vi "_layoutVirtual.vi"(0 "reference":refnum<class "SequenceDiagramGraph.lvclass">, 1 "graphics":refnum<class "Graphics.lvclass">, 2 "grid":refnum<class "Grid.lvclass">, 5 "error in (no error)":errorcluster) -> (14 "reference out":refnum<class "SequenceDiagramGraph.lvclass">, 19 "error out":errorcluster)   [LabVIEW 2012, in "SequenceDiagramGraph.lvclass"]
doc: "public void layoutVirtual(Graphics2D g2, Grid grid)"
uses:
  <resource>/Framework/Providers/Open_GDS/UML/SequenceDiagramGraph_class/SequenceDiagramGraph.lvclass
  <resource>/Framework/Providers/Open_GDS/UML/Graphics_class/Graphics.lvclass
  <resource>/Framework/Providers/Open_GDS/UML/Grid_class/Grid.lvclass
  <resource>/Framework/Providers/Open_GDS/UML/CallNode_class/CallNode.lvclass
  <resource>/Framework/Providers/Open_GDS/UML/AbstractNode_class/AbstractNode.lvclass
  <resource>/Framework/Providers/Open_GDS/UML/AbstractEdge_class/AbstractEdge.lvclass
  <resource>/Framework/Providers/Open_GDS/UML/CallEdge_class/CallEdge.lvclass
  <resource>/Framework/Providers/Open_GDS/UML/ImplicitParameterNode_class/ImplicitParameterNode.lvclass
  <resource>/Framework/Providers/Open_GDS/UML/RectangularNode_class/RectangularNode.lvclass
  <resource>/Framework/Providers/Open_GDS/UML/Graph_class/Graph.lvclass
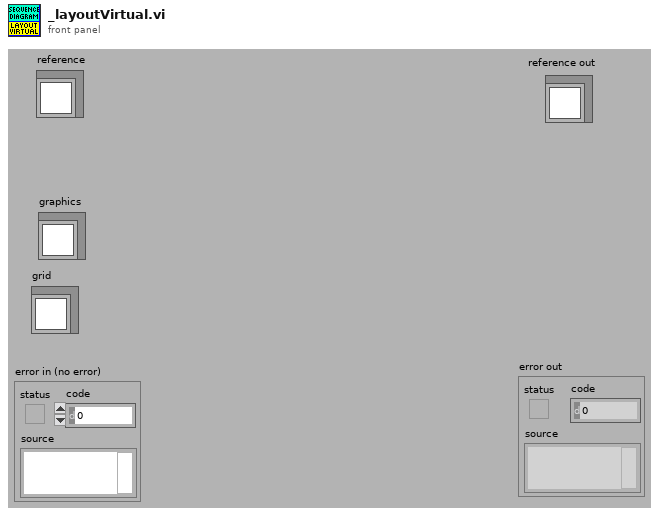
[diagram p1: front panel]
types:
  T1 = typedef "SequenceDiagramGraph.lvclass/ObjectAttributes.ctl" = cluster{"Base class":T2, "none":bool}
  T2 = typedef "Graph.lvclass/ObjectAttributes.ctl" = cluster{"nodes":refnum<class "AbstractNode.lvclass">[], "edges":refnum<class "AbstractEdge.lvclass">[], "nodesToBeRemoved":refnum<class "AbstractNode.lvclass">[], "edgesToBeRemoved":refnum<class "AbstractEdge.lvclass">[], "needsLayout":bool, "LayoutNodes":refnum<class "AbstractNode.lvclass">[]}
  T3 = typedef "Rectangle Rectangle2D.ctl" = cluster{"x":dbl, "y":dbl, "width":dbl, "height":dbl}
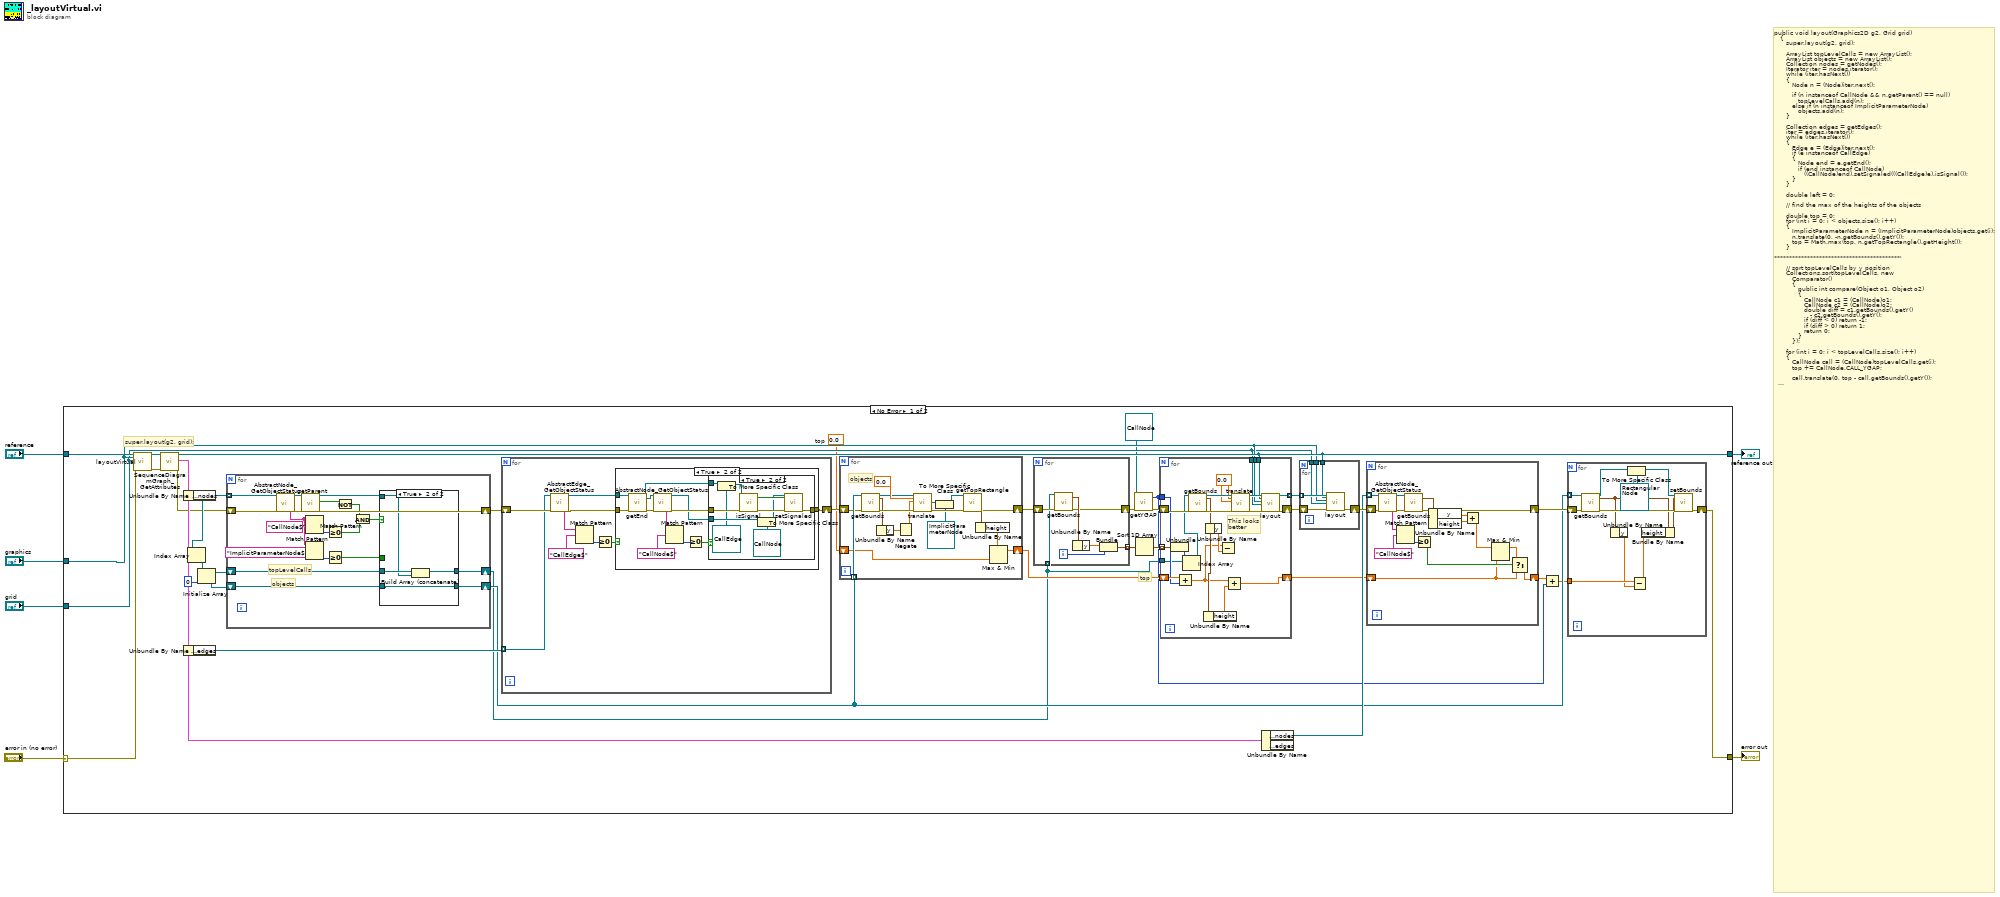
[diagram p0: block diagram]
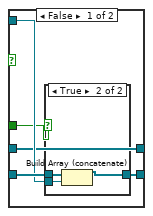
[diagram p4: hidden frame]
diagram:
  # "public void layout(Graphics2D g2, Grid grid)\n   {\n      super.layout(g2, grid);\n\n      ArrayList topLevelCalls = new ArrayList();\n      ArrayList objects = new ArrayList();\n      Collection nodes = getNodes();\n      Iterator iter = nodes.iterator();\n      while (iter.hasNext())\n      {\n         Node n = (Node)iter.next();\n         \n         if (n instanceof CallNode && n.getParent() == null) \n            topLevelCalls.add(n);\n         else if (n instanceof ImplicitParameterNode)\n            objects.add(n);      \n      }\n\n      Collection edges = getEdges();\n      iter = edges.iterator();\n      while (iter.hasNext())\n      {\n         Edge e = (Edge)iter.next();\n         if (e instanceof CallEdge)\n         {\n            Node end = e.getEnd();\n            if (end instanceof CallNode)\n               ((CallNode)end).setSignaled(((CallEdge)e).isSignal());\n         }\n      }\n\n      double left = 0;\n\n      // find the max of the heights of the objects\n\n      double top = 0;\n      for (int i = 0; i < objects.size(); i++)\n      {\n         ImplicitParameterNode n = (ImplicitParameterNode)objects.get(i);\n         n.translate(0, -n.getBounds().getY());\n         top = Math.max(top, n.getTopRectangle().getHeight());\n      }\n\n******************************************'\n\n      // sort topLevelCalls by y position \n      Collections.sort(topLevelCalls, new\n         Comparator()\n         {\n            public int compare(Object o1, Object o2)\n            {\n               CallNode c1 = (CallNode)o1;\n               CallNode c2 = (CallNode)o2;\n               double diff = c1.getBounds().getY()\n                  - c2.getBounds().getY();\n               if (diff < 0) return -1;\n               if (diff > 0) return 1;\n               return 0;\n            }            \n         });\n\n      for (int i = 0; i < topLevelCalls.size(); i++)\n      {\n         CallNode call = (CallNode)topLevelCalls.get(i);\n         top += CallNode.CALL_YGAP;\n\n         call.translate(0, top - call.getBounds().getY());\n         call.layout(this, g2, grid);\n         top += call.getBounds().getHeight();\n      }\n      */\n\n      for (int i = 0; i < topLevelCalls.size(); i++)\n      {\n         CallNode call = (CallNode)topLevelCalls.get(i);\n         call.layout(this, g2, grid);\n      }\n\n      iter = nodes.iterator();\n      while (iter.hasNext())\n      {\n         Node n = (Node)iter.next();\n         if (n instanceof CallNode)\n            top = Math.max(top, n.getBounds().getY()\n               + n.getBounds().getHeight());\n      }\n\n      top += CallNode.CALL_YGAP;\n\n      for (int i = 0; i < objects.size(); i++)\n      {\n         ImplicitParameterNode n = (ImplicitParameterNode)objects.get(i);\n         Rectangle2D b = n.getBounds();\n         n.setBounds(new Rectangle2D.Double(\n            b.getX(), b.getY(), \n            b.getWidth(), top - b.getY()));         \n      }\n   }"
  n1 = case shown="No Error" "error in (no error)" {
    selector: "error in (no error)" -> [w39 w189]
    tunnel: "reference" -> [w42 w190]
    tunnel: [w41 w189] -> w5
    tunnel: [w40 w190] -> w4
    tunnel: "graphics" -> [w38 _]
    tunnel: "grid" -> [w37 _]
    frame No Error {
      w27 = 0.0  # top
      # "top"
      # "super.layout(g2, grid);"
      n2 = call <resource>:"layoutVirtual.vi"("reference"=w42, "graphics"=w38, "grid"=w37, "error in (no error)"=w39) -> ("reference out"=w35:refnum<class "SequenceDiagramGraph.lvclass">, "error out"=w10:errorcluster)  [unwired: 14 out]
      n3 = call <resource>:"SequenceDiagramGraph_GetAttributes.vi"("reference in"=w35, "error in (no error)"=w10) -> ("reference out"=w40:refnum<class "SequenceDiagramGraph.lvclass">, "Attributes"=w36:T1, "error out"=w9:errorcluster)  [unwired: 15 out]
      n4 = Unbundle By Name(w36) -> ("Base class.nodes"=w34:refnum<class "AbstractNode.lvclass">[])
      n5 = Unbundle By Name(w36) -> ("Base class.edges"=w29:refnum<class "AbstractEdge.lvclass">[])
      n6 = Index Array(array=w34) -> (element=w33:refnum<class "AbstractNode.lvclass">)  [unwired: 1 in]
      n7 = Initialize Array(w33, 0 ("dimension size")) -> (w31:refnum<class "AbstractNode.lvclass">[])
      n8 = for {
        tunnel: w34 -> [w95] mode=indexing
        shift-right: [w89] -> w30
        shift-left: w9 -> [w94]
        shift-right: [w90] -> w8
        shift-left: w31 -> [w93]
        shift-right: [w91] -> w12
        shift-left: w31 -> [w92]
        # "objects"
        # "topLevelCalls"
        n9 = call <resource>:"AbstractNode_GetObjectStatus.vi"("reference in"=w95, "error in (no error)"=w94) -> ("Class name"=w79:string, "reference out"=w85:refnum<class "AbstractNode.lvclass">, "error out"=w84:errorcluster)  [unwired: 15 out]
        n10 = call-dynamic "getParent.vi"("reference"=w85, "error in (no error)"=w84) -> ("reference out"=w82:refnum<class "AbstractNode.lvclass">, "ValidParent"=w77:bool, "error out"=w89:errorcluster)  [unwired: 13 in, 2 out]
        n11 = Match Pattern(string=w79, regular expression="CallNode$") -> (offset past match=w87:i32)  [unwired: 4 out]
        n12 = Match Pattern(string=w79, regular expression="ImplicitParameterNode$") -> (offset past match=w80:i32)  [unwired: 4 out]
        n13 = Greater Or Equal To 0?(x=w87) -> (x >= 0?=w88:bool)
        n14 = Greater Or Equal To 0?(x=w80) -> (x >= 0?=w78:bool)
        n15 = Not(x=w77) -> (.not. x?=w76:bool)
        n16 = And(x=w76, y=w88) -> (x .and. y?=w83:bool)
        n17 = case shown="True" w83 {
          tunnel: w93 -> [w97 w108]
          tunnel: w92 -> [w100 w105]
          tunnel: w82 -> [w99 w107]
          tunnel: [w98 w105] -> w91
          tunnel: [w97 w106] -> w90
          tunnel: w78 -> [w96 _]
          frame False {
            n18 = case shown="True" w96 {
              tunnel: w100 -> [w101 w104]
              tunnel: w99 -> [_ w103]
              tunnel: [w101 w102] -> w98
              frame False {
              }
              frame True {
                n19 = Build Array (concatenate)(w104, w103) -> (w102:refnum<class "AbstractNode.lvclass">[])
              }
            }
          }
          frame True {
            n20 = Build Array (concatenate)(w108, w107) -> (w106:refnum<class "AbstractNode.lvclass">[])
          }
        }
      }
      n21 = for {
        shift-right: [w50] -> w28
        shift-left: w30 -> [w51]
        tunnel: w29 -> [w49] mode=indexing
        n22 = call <resource>:"AbstractEdge_GetObjectStatus.vi"("reference in"=w49, "error in (no error)"=w51) -> ("Class name"=w46:string, "reference out"=w44:refnum<class "AbstractEdge.lvclass">, "error out"=w43:errorcluster)  [unwired: 15 out]
        n23 = Match Pattern(string=w46, regular expression="CallEdge$") -> (offset past match=w47:i32)  [unwired: 4 out]
        n24 = Greater Or Equal To 0?(x=w47) -> (x >= 0?=w45:bool)
        n25 = case shown="True" w45 {
          tunnel: w44 -> [_ w64]
          tunnel: w43 -> [w52 w63]
          tunnel: [w52 w53] -> w50
          frame False {
          }
          frame True {
            n26 = call-dynamic "getEnd.vi"("reference"=w64, "error in (no error)"=w63) -> ("reference out"=w55:refnum<class "AbstractEdge.lvclass">, "endNode"=w60:refnum<class "AbstractNode.lvclass">, "error out"=w59:errorcluster)  [unwired: 14 in, 1 out]
            n27 = call <resource>:"AbstractNode_GetObjectStatus.vi"("reference in"=w60, "error in (no error)"=w59) -> ("Class name"=w58:string, "reference out"=w54:refnum<class "AbstractNode.lvclass">, "error out"=w56:errorcluster)  [unwired: 15 out]
            n28 = Match Pattern(string=w58, regular expression="CallNode$") -> (offset past match=w62:i32)  [unwired: 4 out]
            n29 = Greater Or Equal To 0?(x=w62) -> (x >= 0?=w57:bool)
            n30 = case shown="True" w57 {
              tunnel: w56 -> [w65 w75]
              tunnel: w55 -> [_ w68]
              tunnel: w54 -> [_ w71]
              tunnel: [w65 w72] -> w53
              frame False {
              }
              frame True {
                n31 = To More Specific Class(target class=refnum<class "CallEdge.lvclass"> refnum ("reference"), reference=w68) -> (specific class reference=w66:refnum<class "CallEdge.lvclass">)  [unwired: 1 in, 1 out]
                n32 = call-dynamic "isSignal.vi"("reference"=w66, "error in (no error)"=w75) -> ("signal"=w74:bool, "error out"=w73:errorcluster)  [unwired: 15 in, 1 out]
                n33 = To More Specific Class(target class=refnum<class "CallNode.lvclass"> refnum ("reference"), reference=w71) -> (specific class reference=w69:refnum<class "CallNode.lvclass">)  [unwired: 1 in, 1 out]
                n34 = call-dynamic "setSignaled.vi"("reference"=w69, "signal"=w74, "error in (no error)"=w73) -> ("error out"=w72:errorcluster)  [unwired: 15 in, 1 out]
              }
            }
          }
        }
      }
      n35 = for {
        shift-right: [w175] -> w26
        shift-left: w28 -> [w184]
        tunnel: w12 -> [w187] mode=indexing
        shift-right: [w180] -> w23
        shift-left: w27 -> [w177]
        # "objects"
        n36 = call-dynamic "getBounds.vi"("reference"=w187, "error in (no error)"=w184) -> ("reference out"=w186:refnum<class "AbstractNode.lvclass">, "bounds"=w183:T3, "error out"=w185:errorcluster)  [unwired: 15 in]
        n37 = Unbundle By Name(w183) -> ("y"=w182:dbl)
        n38 = Negate(x=w182) -> (-x=w181:dbl)
        n39 = call-dynamic "translate.vi"("reference"=w186, "dx"=0.0, "dy"=w181, "error in (no error)"=w185) -> ("reference out"=w173:refnum<class "AbstractNode.lvclass">, "error out"=w179:errorcluster)  [unwired: 14 in]
        n40 = To More Specific Class(target class=refnum<class "ImplicitParameterNode.lvclass"> refnum ("reference"), reference=w173) -> (specific class reference=w172:refnum<class "ImplicitParameterNode.lvclass">)  [unwired: 1 in, 1 out]
        n41 = call-dynamic "getTopRectangle.vi"("reference"=w172, "error in (no error)"=w179) -> ("bounds"=w178:T3, "error out"=w175:errorcluster)  [unwired: 15 in, 1 out]
        n42 = Unbundle By Name(w178) -> ("height"=w176:dbl)
        n43 = Max & Min(x=w176, y=w177) -> (max(x,y)=w180:dbl)  [unwired: 1 out]
      }
      n44 = for {
        tunnel: w8 -> [w168] mode=indexing
        shift-right: [w166] -> w22
        shift-left: w26 -> [w171]
        tunnel: [w167] -> w25 mode=indexing
        i -> [w165]
        n45 = call-dynamic "getBounds.vi"("reference"=w168, "error in (no error)"=w171) -> ("bounds"=w170:T3, "error out"=w166:errorcluster)  [unwired: 15 in, 1 out]
        n46 = Unbundle By Name(w170) -> ("y"=w169:dbl)
        n47 = Bundle("y"=w169, w165) -> (w167:cluster{"y":dbl, i32})  [unwired: 1 out]
      }
      n48 = call <resource>:"getYGAP.vi"("reference"=refnum<class "CallNode.lvclass"> refnum, "error in (no error)"=w22) -> ("CALL_YGAP"=w14:i32, "error out"=w21:errorcluster)  [unwired: 16 out]
      n49 = Sort 1D Array(array=w25) -> (sorted array=w24:cluster{"y":dbl, i32}[])
      n50 = for {
        tunnel: w24 -> [w164] mode=indexing
        shift-right: [w148] -> w16
        shift-left: w23 -> [w153]
        tunnel: w40 -> [w158]
        tunnel: w38 -> [w157]
        tunnel: w37 -> [w156]
        shift-right: [w155] -> w20
        shift-left: w21 -> [w163]
        tunnel: w14 -> [w152]
        tunnel: [w147] -> w19 mode=indexing
        tunnel: w8 -> [w145]
        w146 = 0.0 ("dx")
        # "This looks\nbetter"
        n51 = Unbundle(w164) -> (w144:i32)  [unwired: 1 out]
        n52 = Add(x=w153, y=w152) -> (x+y=w150:dbl)
        n53 = Index Array(array=w145, index=w144) -> (element=w143:refnum<class "AbstractNode.lvclass">)
        n54 = call-dynamic "getBounds.vi"("reference"=w143, "error in (no error)"=w163) -> ("reference out"=w162:refnum<class "AbstractNode.lvclass">, "bounds"=w154:T3, "error out"=w161:errorcluster)  [unwired: 15 in]
        n55 = Unbundle By Name(w154) -> ("height"=w149:dbl)
        n56 = Unbundle By Name(w154) -> ("y"=w151:dbl)
        n57 = Subtract(x=w150, y=w151) -> ()  [unwired: 1 out]
        n58 = Add(x=w150, y=w149) -> (x+y=w148:dbl)
        n59 = call-dynamic "translate.vi"("reference"=w162, "dx"=w146, "dy"=w146, "error in (no error)"=w161) -> ("reference out"=w160:refnum<class "AbstractNode.lvclass">, "error out"=w159:errorcluster)  [unwired: 14 in]
        n60 = call-dynamic "layout.vi"("reference"=w160, "graph"=w158, "graphics"=w157, "grid"=w156, "error in (no error)"=w159) -> ("reference out"=w147:refnum<class "AbstractNode.lvclass">, "error out"=w155:errorcluster)  [unwired: 13 in]
      }
      n61 = Unbundle By Name(w36) -> ("Base class.nodes"=w17:refnum<class "AbstractNode.lvclass">[])  [unwired: 1 out]
      n62 = for {
        shift-right: [w137] -> w18
        shift-left: w20 -> [w142]
        tunnel: w40 -> [w140]
        tunnel: w19 -> [w141] mode=indexing
        tunnel: w38 -> [w139]
        tunnel: w37 -> [w138]
        n63 = call-dynamic "layout.vi"("reference"=w141, "graph"=w140, "graphics"=w139, "grid"=w138, "error in (no error)"=w142) -> ("error out"=w137:errorcluster)  [unwired: 13 in, 1 out]
      }
      n64 = for {
        shift-right: [w121] -> w13
        shift-left: w18 -> [w133]
        tunnel: w17 -> [w132] mode=indexing
        shift-right: [w130] -> w15
        shift-left: w16 -> [w126]
        n65 = call <resource>:"AbstractNode_GetObjectStatus.vi"("reference in"=w132, "error in (no error)"=w133) -> ("Class name"=w134:string, "reference out"=w129:refnum<class "AbstractNode.lvclass">, "error out"=w128:errorcluster)  [unwired: 15 out]
        n66 = Match Pattern(string=w134, regular expression="CallNode$") -> (offset past match=w136:i32)  [unwired: 4 out]
        n67 = call-dynamic "getBounds.vi"("reference"=w129, "error in (no error)"=w128) -> ("bounds"=w127:T3, "error out"=w121:errorcluster)  [unwired: 15 in, 1 out]
        n68 = Greater Or Equal To 0?(x=w136) -> (x >= 0?=w131:bool)
        n69 = Unbundle By Name(w127) -> ("y"=w124:dbl, "height"=w123:dbl)
        n70 = Add(x=w124, y=w123) -> (x+y=w122:dbl)
        n71 = Max & Min(x=w122, y=w126) -> (max(x,y)=w125:dbl)  [unwired: 1 out]
        n72 = Select(t=w125, s=w131, f=w126) -> (s? t:f=w130:dbl)
      }
      n73 = Add(x=w15, y=w14) -> (x+y=w11:dbl)
      n74 = for {
        shift-right: [w117] -> w41
        shift-left: w13 -> [w120]
        tunnel: w12 -> [w119] mode=indexing
        tunnel: w11 -> [w114]
        n75 = call-dynamic "getBounds.vi"("reference"=w119, "error in (no error)"=w120) -> ("reference out"=w111:refnum<class "AbstractNode.lvclass">, "bounds"=w116:T3, "error out"=w118:errorcluster)  [unwired: 15 in]
        n76 = Unbundle By Name(w116) -> ("y"=w113:dbl)
        n77 = To More Specific Class(target class=refnum<class "RectangularNode.lvclass"> refnum ("reference"), reference=w111) -> (specific class reference=w109:refnum<class "RectangularNode.lvclass">)  [unwired: 1 in, 1 out]
        n78 = Subtract(x=w114, y=w113) -> (x-y=w112:dbl)
        n79 = Bundle By Name(cluster=w116, "height"=w112) -> (w115:T3)
        n80 = call-dynamic "setBounds.vi"("reference"=w109, "bounds"=w115, "error in (no error)"=w118) -> ("error out"=w117:errorcluster)  [unwired: 15 in, 1 out]
      }
    }
    frame Error {
    }
  }
  "reference out" <- w4
  "error out" <- w5
